vi "Create FPGA Addon.vi"(7 "Configuration (.dat)":path, 8 "error in (no error)":errorcluster, 9 "RIO Device (Use Config if Empty)":string, 10 "Name":string, 11 "Custom Devices Ref":refnum<k24>) -> (0 "error out":errorcluster, 3 "Custom Devices Ref":refnum<k24>)   [LabVIEW 2019, in "FPGA Addon SysDef API.lvlib"]
uses:
  FPGA Addon SysDef API.lvlib
  NationalInstruments.VeriStand.SystemDefinitionAPI
  Shared/Constants.vi
  <vilib>/NI/NI VeriStand Advanced SysDef API/_SubVIs/SysDef.Property.Set.String.vi
  <vilib>/NI/NI VeriStand Custom Device Import and Export Tool/ImportExport.lvlib
  Shared/FPGA Addon Shared.lvlib
  <vilib>/NI/NI VeriStand Advanced SysDef API/SysDef API/Advanced System Definition.lvlib
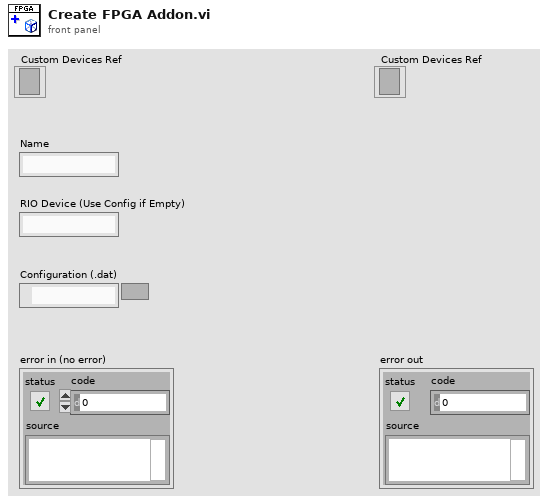
[diagram p1: front panel]
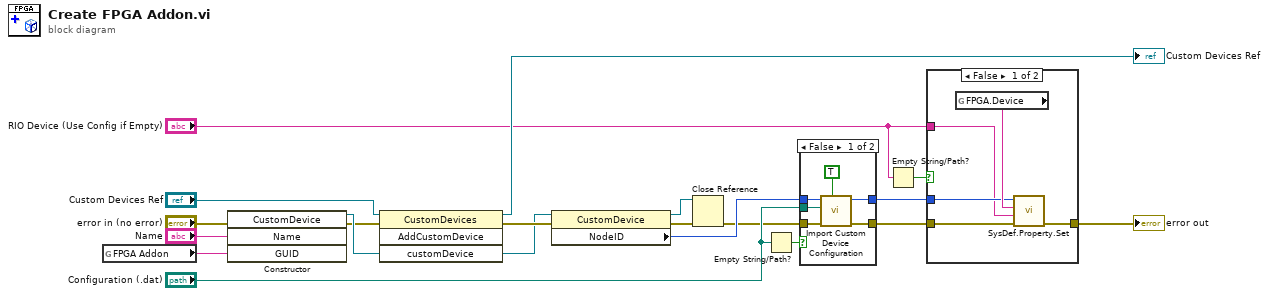
[diagram p0: block diagram]
diagram:
  n1 = global read "Constants.vi" "FPGA Addon"() -> (w14:string)
  n2 = constructor class="CustomDevice"(error in="error in (no error)", "Name"="Name", "GUID"=w14) -> (reference out=w10:refnum<k24>, error out=w9:errorcluster)  [unwired: 2 in, 3 out]
  n3 = invoke class="CustomDevices" method="AddCustomDevice"(reference="Custom Devices Ref", error in=w9, "customDevice"=w10) -> (reference out=→"Custom Devices Ref":refnum<k24>, error out=w19:errorcluster)  [unwired: 1 in, 2 out]
  n4 = property class="CustomDevice"(reference=w10, error in=w19) -> (reference out=w17:refnum<k24>, error out=w18:errorcluster, "NodeID"=w7:u64)
  n5 = Close Reference(reference=w17, error in (no error)=w18) -> (error out=w6:errorcluster)
  n6 = Empty String/Path?(string/path="Configuration (.dat)") -> (empty?=w15:bool)
  n7 = case shown="False" w15 {
    tunnel: [w25 w27] -> w4
    tunnel: w6 -> [w24 w27]
    tunnel: w7 -> [w23 w26]
    tunnel: "Configuration (.dat)" -> [w22 _]
    tunnel: [w20 w26] -> w1
    frame False {
      n8 = call <vilib>:"Import Custom Device Configuration.vi"("Overwrite Existing?"=TRUE, "error in (no error)"=w24, "Path"=w22, "NodeID"=w23) -> ("error out"=w25:errorcluster, "NodeID out"=w20:u64)  [unwired: 5 in, 1 out]
    }
    frame True {
    }
  }
  n9 = Empty String/Path?(string/path="RIO Device (Use Config if Empty)") -> (empty?=w8:bool)
  n10 = case shown="False" w8 {
    tunnel: w4 -> [w32 w33]
    tunnel: [w31 w33] -> w3
    tunnel: w1 -> [w29 _]
    tunnel: "RIO Device (Use Config if Empty)" -> [w28 _]
    frame False {
      n11 = global read "Constants.vi" "FPGA.Device"() -> (w30:string)
      n12 = call-poly <vilib>:"SysDef.Property.Set.vi"("error in (no error)"=w32, "Value"=w28, "Property Name"=w30, "nodeID"=w29) -> ("error out"=w31:errorcluster)  [unwired: 6 in, 1 out]
    }
    frame True {
    }
  }
  "error out" <- w3
